vi "TestMotionControl.vi"() -> ()   [LabVIEW 2016]
uses:
  <vilib>/Platform/TimedLoop/XDataNode/XDataNode.xnode
  <vilib>/Platform/TimedLoop/XDataNode/nitl_modes.ctl
  <vilib>/Platform/TimedLoop/XDataNode/XDNodeRunTimeDep.lvlib
  <vilib>/Platform/TimedLoop/XDataNode/wakeup.ctl
  <vilib>/Platform/TimedLoop/XDataNode/timing_clust.ctl
  <vilib>/robotics/Steering/Steering Frame/NI_Robotics_Steering Frame.lvclass
  <vilib>/robotics/Steering/Steering Frame/Apply Steering Frame Velocity to Wheels.vi
  <vilib>/myRIO/Instrument Drivers/Utilities/Utilities.lvlib
  <vilib>/robotics/Steering/Differential Steering Frame/NI_Robotics_Differential Steering Frame.lvclass
  C:/Program Files (x86)/National Instruments/LabVIEW 2016/vi.lib/robotics/Steering/Special Steering Frame/NI_Robotics_Special Steering Frame.lvclass
  C:/Program Files (x86)/National Instruments/LabVIEW 2016/vi.lib/robotics/Steering/Steering Frame/NI_Robotics_Steering Frame.lvclass
  <vilib>/robotics/Steering/Wheel/Rotation Direction.ctl
  <vilib>/robotics/Steering/Wheel/NI_Robotics_Wheel.lvclass
  <vilib>/robotics/Steering/Wheel/Wheel Parameters.ctl
  MotorControl/Configurations.ctl
panel:
  out "Heading Frame":cluster{"X":sgl, "Y":sgl, "theta":dbl}
  out "Robot Position":cluster{dbl[], dbl[]}(graph)
  in  "stop":bool
  out "Current State":string="Next Goal"
  in  "Start!":bool
  out "Frame Velocity":dbl[](array[numeric])
  in  "Robot Configuration":T1={"wheel parameters"={"wheel radius"=0.05, "gear ratio"=1.0, "forward rotation direction"=0}, "wheel separation"=0.19, "Encoder Pulse Per Rev"=1856.0, "Update Period (sec)"=0.02, "Initial posture frame"=[0.0, 0.0, 0.0]} {"wheel parameters"."forward rotation direction" items=["Clockwise", "Counterclockwise"]}
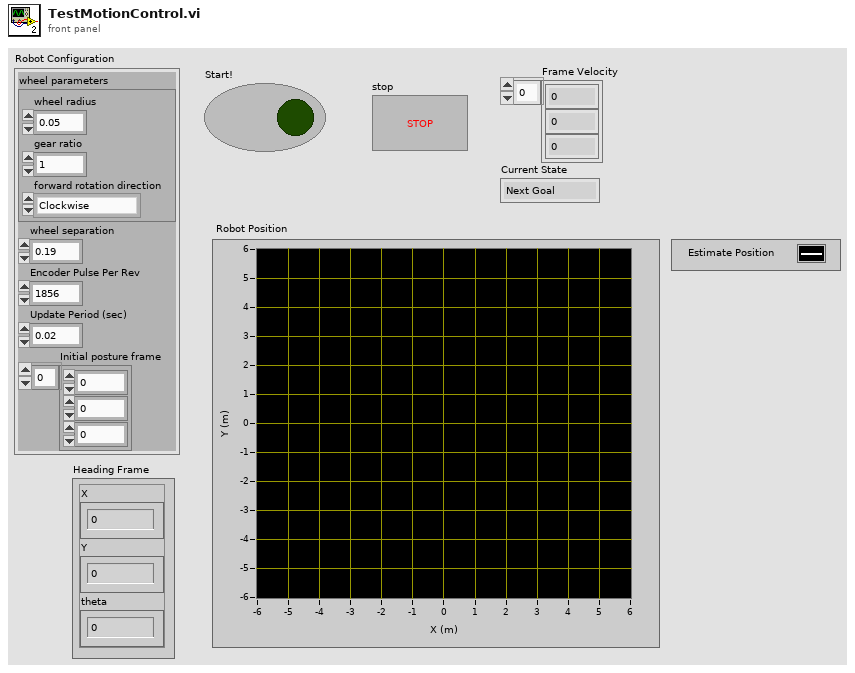
[diagram p1: front panel]
types:
  T1 = typedef "Configurations.ctl" = cluster{"wheel parameters":T2, "wheel separation":dbl, "Encoder Pulse Per Rev":dbl, "Update Period (sec)":dbl, "Initial posture frame":dbl[]}
  T2 = typedef "NI_Robotics_Wheel.lvclass/Wheel Parameters.ctl" = cluster{"wheel radius":dbl, "gear ratio":dbl, "forward rotation direction":T3}
  T3 = typedef "NI_Robotics_Wheel.lvclass/Rotation Direction.ctl" = u16
  T4 = typedef "MotorObject.ctl" = cluster{"PWM Motor Left":T5, "PWM Motor Right":T5, "DIR Motor Left":T12, "Encoder Motor Left":T15, "Encoder Motor Right":T15, "DIR Motor Right":T12, "Left DIR Forward":bool}
  T5 = typedef "PWM.lvlib/PWM Reference.ctl" = cluster{"myRIO Reference":T6, "PWM Channels Enum":T10, "PWM Configuration":T11}
  T6 = typedef "myRIO Generic Hardware Reference.ctl" = cluster{"myRIO Model":T7, "myRIO Hardware Reference":T8}
  T7 = typedef "Hardware Version Enum.ctl" = enum16{"Unknown", "myRIO-1900", "myRIO-1950", "roboRIO", "NI ELVIS RIO CM"}
  T8 = typedef "myRIO v1.0 Reference.ctl" = cluster{"Generic FPGA Reference":T9, "Allow multiple opens":bool}
  T9 = typedef "Generic FPGA Reference.ctl" = refnum<k20>
  T10 = typedef "PWM Channels Enum.ctl" = enum16{"Not Connected", "C/PWM0", "C/PWM1", "A/PWM0", "A/PWM1", "A/PWM2", "B/PWM0", "B/PWM1", "B/PWM2", "PWM/PWM0", "PWM/PWM1", "PWM/PWM2", "PWM/PWM3", "PWM/PWM4", "PWM/PWM5", "PWM/PWM6", "PWM/PWM7", "PWM/PWM8", "PWM/PWM9"}
  T11 = typedef "PWM.lvlib/PWM Configuration.ctl" = cluster{"Frequency":dbl, "Duty Cycle":dbl}
  T12 = typedef "DIO.lvlib/DIO Reference.ctl" = cluster{"myRIO Reference":T6, "DIO Channels List":T13}
  T13 = typedef "DIO Channels List.ctl" = T14[]
  T14 = typedef "DIO Channels Enum.ctl" = enum16{"Not Connected", "C/DIO0", "C/DIO1", "C/DIO2", "C/DIO3", "C/DIO4", "C/DIO5", "C/DIO6", "C/DIO7", "A/DIO0", "A/DIO1", "A/DIO2", "A/DIO3", "A/DIO4", "A/DIO5", "A/DIO6", "A/DIO7", "A/DIO8", "A/DIO9", "A/DIO10", "A/DIO11", "A/DIO12", "A/DIO13", "A/DIO14", "A/DIO15", "B/DIO0", "B/DIO1", "B/DIO2", "B/DIO3", "B/DIO4", "B/DIO5", "B/DIO6", "B/DIO7", "B/DIO8", "B/DIO9", "B/DIO10", "B/DIO11", "B/DIO12", "B/DIO13", "B/DIO14", "B/DIO15", "LED0", "LED1", "LED2", "LED3", "Button0", "DIO/DIO0", "DIO/DIO1", "DIO/DIO2", "DIO/DIO3", "DIO/DIO4", "DIO/DIO5", "DIO/DIO6", "DIO/DIO7", "DIO/DIO8", "DIO/DIO9", "SPI/CS0", "SPI/CS1", "SPI/CS2", "SPI/CS3", "LED RADIO (Green)", "LED RADIO (Red)", "LED COMM (Green)", "LED COMM (Red)", "LED MODE (Green)", "LED MODE (Red)"}
  T15 = typedef "Encoder.lvlib/Encoder Reference.ctl" = cluster{"myRIO Reference":T6, "Encoder Channels Enum":T16}
  T16 = typedef "Encoder Channels Enum.ctl" = enum16{"Not Connected", "C/ENC0", "C/ENC1", "A/ENC", "B/ENC", "DIO/ENC0", "DIO/ENC1", "DIO/ENC2", "DIO/ENC3", "DIO/ENC4"}
  T17 = typedef "XDNodeRunTimeDep.lvlib/timing_clust.ctl" = cluster{"Expected End [f-1]":u64, "Actual End [f-1]":u64, "Finished Late? [f-1]":bool, "Expected End [i-1]":u64, "Actual End [i-1]":u64, "Finished Late? [i-1]":bool, "Expected Start [i]":u64, "Actual Start [i]":u64, "Expected Start [f]":u64, "Actual Start [f]":u64, "Source Name":string, "Structure Name":string, "Period":i64, "Deadline":i64, "Offset":i64, "Start":i64, "Priority":i32, "Timeout":i32, "Mode":T18, "Wakeup Reason":T19, "Error":errorcluster, "Source Type":string, "Secondary Source Type":string, "Global End Time":u64, "Global Start Time":u64, "Frame Duration":u64, "Iteration Duration":u64, "Assigned CPU":i32, "I/O Scan Engine Mode":u32}
  T18 = typedef "XDNodeRunTimeDep.lvlib/nitl_modes.ctl" = enum32{"No Change", "Process missed periods, maintain original phase", "Discard missed periods, maintain original phase", "Process missed periods, ignore original phase", "Discard missed periods, ignore original phase"}
  T19 = typedef "XDNodeRunTimeDep.lvlib/wakeup.ctl" = enum32{"Normal", "Aborted", "Asynchronous wakeup", "Timing source error", "Timed loop error", "Timeout"}
  T20 = cluster{"Left Rad Per Sec":dbl, "Right Rad Per Sec":dbl, "Left Pulse Per Sec":dbl, "Right Pulse Per Sec":dbl}
  T21 = typedef "NI_Robotics_Wheel.lvclass/Wheel State.ctl" = cluster{"wheel name":string, "forward angular velocity":dbl, "caster angular velocity":dbl, "caster wheel angle (rad)":dbl, "steering angle (rad)":dbl}
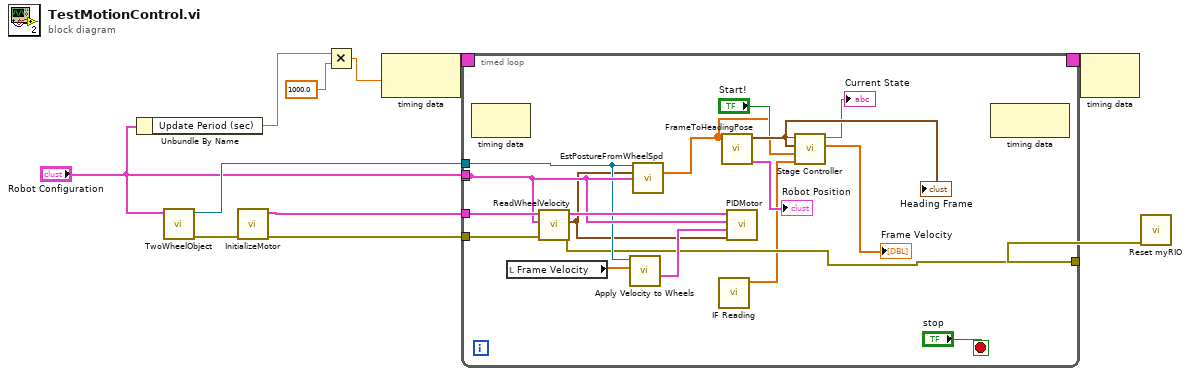
[diagram p0: block diagram]
diagram:
  n1 = Unbundle By Name("Robot Configuration") -> ("Update Period (sec)"=w4:dbl)
  n2 = call "TwoWheelObject.vi"("Robot Configuration"="Robot Configuration") -> ("error out"=w11:errorcluster, "differential steering frame out"=w3:refnum<class "NI_Robotics_Differential Steering Frame.lvclass">)  [unwired: 9 in]
  n3 = call "InitializeMotor.vi"("error in"=w11) -> ("error out"=w7:errorcluster, "Motor Ref"=w8:T4)  [unwired: 9 in]
  n4 = Multiply(x=w4, y=1000.0) -> (x*y=w5:dbl)
  n5 = node-c288(w5) -> (w10:T17)
  n6 = timed-loop {
    timing: w10 -> [_]
    timing-out: [_] -> w9
    tunnel: w8 -> [w28]
    tunnel: w7 -> [w27]
    tunnel: w3 -> [w19]
    tunnel: [w25] -> _
    tunnel: "Robot Configuration" -> [w25]
    tunnel: [w16] -> w1
    stop <- "stop" stop-if-true
    n7 = node-c288() -> ()  [unwired: 1 in, 1 out]
    n8 = local read "Frame Velocity"() -> (w20:dbl[])
    n9 = call "ReadWheelVelocity.vi"("error in"=w27, "Robot Configuration"=w25, "Motor Ref"=w28) -> ("error out"=w16:errorcluster, "Wheel Velocity"=w14:T20, "Motor Ref"=w26:T4)  [unwired: 6 in]
    n10 = call-poly <vilib>:"Apply Velocity to Wheels.vi"("steering frame velocity"=w20, "steering frame in"=w19) -> ("calculated wheel states"=w18:T21[])  [unwired: 6 in, 3 out]
    n11 = call "EstPostureFromWheelSpd.vi"("differential steering frame in"=w19, "Wheel Velocity"=w14, "Robot Configuration"=w25) -> ("estimated steering frame posture"=w13:dbl[])  [unwired: 10 in, 2 out]
    n12 = call "IF Reading.vi"() -> ("IF readings (meters)"=w12:dbl[])  [unwired: 10 in, 1 out]
    n13 = call "FrameToHeadingPose.vi"("Posture In"=w13) -> ("Robot Vector"=→"Robot Position":cluster{"Array":dbl[], "Array":dbl[]}, "Heading Frame"=w23:cluster{"X":sgl, "Y":sgl, "theta":dbl})  [unwired: 7 in, 2 out]
    "Heading Frame" <- w23
    n14 = call "PIDMotor.vi"("Motor Object"=w26, "Robot Configuration"=w25, "calculated wheel states"=w18, "Wheel Velocity"=w14) -> ()  [unwired: 7 in]
    n15 = call "Stage Controller.vi"("Obs Distances Measure Array"=w12, "Posture In"=w13, "Robot Frame (World)"=w23, "Start!"="Start!") -> ("Frame Velocity"=→"Frame Velocity":dbl[], "Current State"=→"Current State":string)  [unwired: 6 in]
    n16 = node-c288() -> ()  [unwired: 1 in, 1 out]
  }
  n17 = node-c288(w9) -> ()  [unwired: 1 out]
  n18 = call <vilib>:"Reset myRIO.vi"("error in (no error)"=w1) -> ()  [unwired: 10 in, 1 out]
